vi "Order_Steps.vi"(0 "System data":T1, 1 "Wash Options":refnum<vi>, 3 "error in (no error)":errorcluster) -> (5 "System data out":T1, 7 "error out":errorcluster)   [LabVIEW 2023]
uses:
  Controls/System_Data.ctl
  Controls/Wash Options.ctl
  Controls/State.ctl
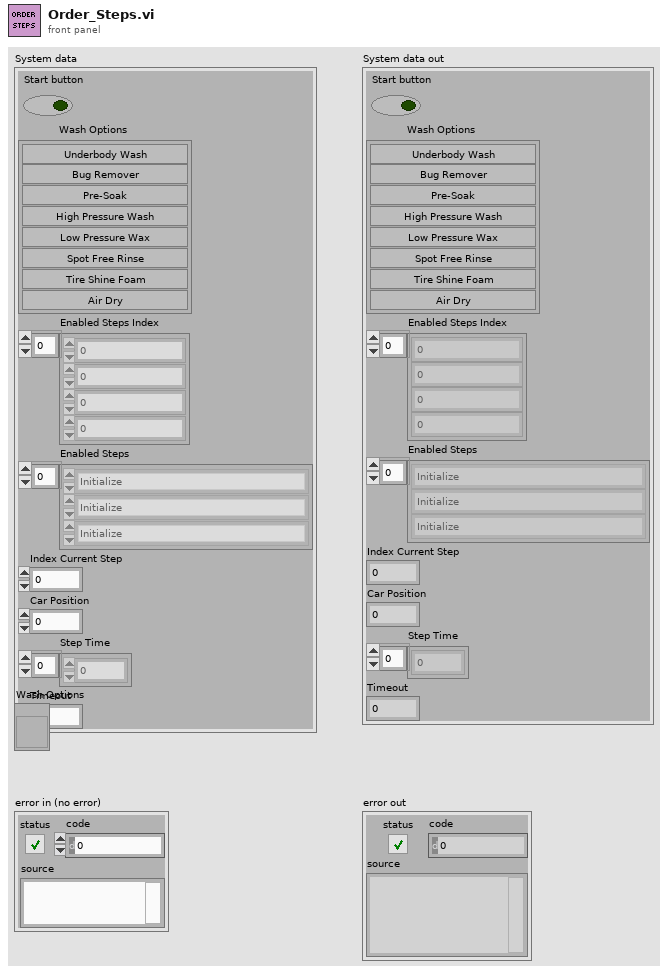
[diagram p1: front panel]
types:
  T1 = typedef "System_Data.ctl" = cluster{"Start button":bool, "Wash Options":T2, "Enabled Steps Index":i32[], "Enabled Steps ":T3[], "Index Current Step":i32, "Car Position":u8, "Step Time":dbl[], "Timeout":i32}
  T2 = typedef "Wash Options.ctl" = cluster{"Underbody Wash":bool, "Bug Remover":bool, "Pre-Soak":bool, "High Pressure Wash":bool, "Low Pressure Wax":bool, "Spot Free Rinse":bool, "Tire Shine Foam":bool, "Air Dry":bool}
  T3 = typedef "State.ctl" = enum16{"Initialize", "Wait for Something", "Step Completed", "Save Wash Options", "Start Process", "Car Position", "Order Steps to follow", "Underbody Wash", "Bug Remover", "Pre-Soak", "High Pressure Wash", "Low Pressure Wax", "Spot Free Rinse", "Tire Shine Foam", "Air Dry", "Vehicle out of position", "Process Complete", "Stop Application"}
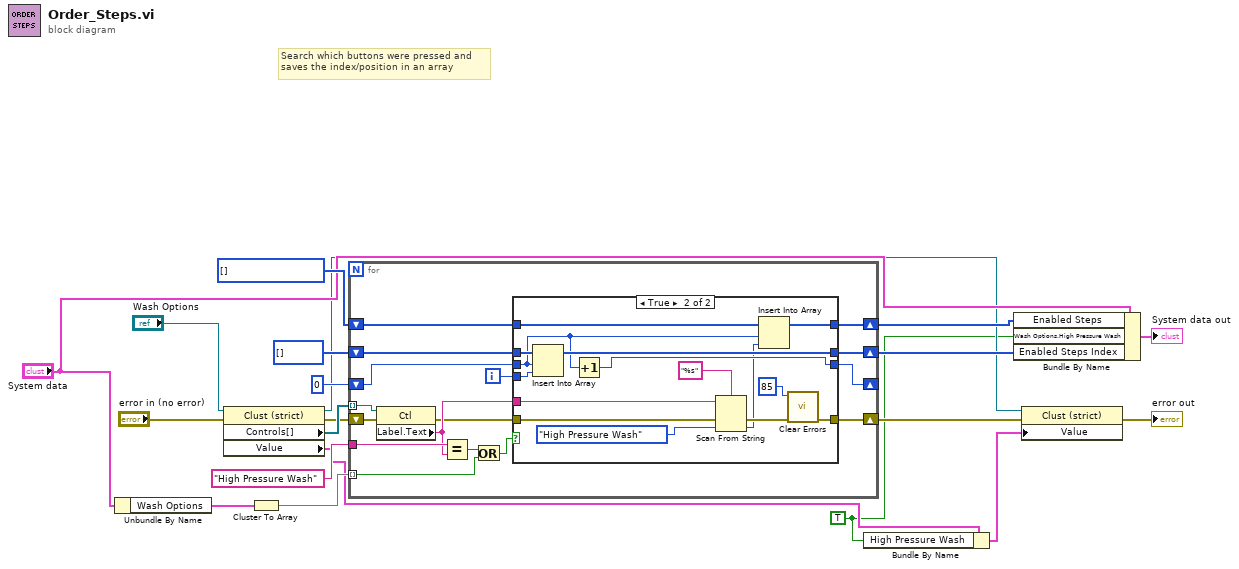
[diagram p0: block diagram]
diagram:
  w9 = T3[] [] items=["Initialize", "Wait for Something", "Step Completed", "Save Wash Options", "Start Process", "Car Position", "Order Steps to follow", "Underbody Wash", "Bug Remover", "Pre-Soak", "High Pressure Wash", "Low Pressure Wax", "Spot Free Rinse", "Tire Shine Foam", "Air Dry", "Vehicle out of position", "Process Complete", "Stop Application"]
  w1 = TRUE ("Wash Options.High Pressure Wash")
  # "Search which buttons were pressed and\nsaves the index/position in an array"
  n1 = Unbundle By Name("System data") -> ("Wash Options"=w20:T2)
  n2 = property class="Clust (strict)"(reference="Wash Options", error in="error in (no error)") -> (reference out=w4:refnum<vi>, error out=w13:errorcluster, "Controls[]"=w14:refnum<vi>[], "Value"=w3:T2)
  n3 = Cluster To Array(cluster=w20) -> (array=w19:bool[])
  n4 = for {
    tunnel: w19 -> [w29] mode=indexing
    shift-right: [w35] -> w8
    shift-left: i32[] [] -> [w36]
    shift-right: [w33] -> _
    shift-left: 0 -> [w34]
    tunnel: w14 -> [w23] mode=indexing
    tunnel: "High Pressure Wash" -> [w26]
    shift-right: [w31] -> w10
    shift-left: w13 -> [w32]
    shift-right: [w28] -> w7
    shift-left: w9 -> [w27]
    i -> [w24]
    n5 = property class="Ctl"(reference=w23, error in=w32) -> (error out=w21:errorcluster, "Label.Text"=w25:string)  [unwired: 1 out]
    n6 = Equal?(x=w26, y=w25) -> (x = y?=w22:bool)
    n7 = Or(x=w22, y=w29) -> (x .or. y?=w30:bool)
    n8 = case shown="True" w30 {
      tunnel: w36 -> [w40 w55]
      tunnel: [w40 w54] -> w35
      tunnel: w34 -> [w39 w45]
      tunnel: [w39 w53] -> w33
      tunnel: w24 -> [_ w52]
      tunnel: w21 -> [w38 w48]
      tunnel: [w38 w42] -> w31
      tunnel: w27 -> [w37 w51]
      tunnel: [w37 w50] -> w28
      tunnel: w25 -> [_ w43]
      frame False {
      }
      frame True {
        n9 = Insert Into Array(array=w55, index=w45, new element=w52) -> (w54:i32[])
        n10 = Increment(x=w45) -> (x+1=w53:i32)
        n11 = Scan From String(format string="%s", input string=w43, error in=w48, default 1=State."High Pressure Wash" ("State")) -> (error out=w47:errorcluster, output 1=w46:T3)  [unwired: 1 in, 2 out]
        n12 = Insert Into Array(array=w51, index=w45, new element=w46) -> (w50:T3[])
        n13 = call <vilib>:"Clear Errors.vi"("error in (no error)"=w47, "specific error code to clear (0: all)"=85) -> ("error out"=w42:errorcluster)  [unwired: 4 in, 1 out]
      }
    }
  }
  n14 = Bundle By Name(cluster=w3, "High Pressure Wash"=w1) -> (w2:T2)
  n15 = Bundle By Name(cluster="System data", "Enabled Steps"=w7, "Wash Options.High Pressure Wash"=w1, "Enabled Steps Index"=w8) -> (→"System data out":T1)
  n16 = property class="Clust (strict)"(reference=w4, error in=w10, "Value"=w2) -> (error out=→"error out":errorcluster)  [unwired: 1 out]
